vi "Main_Stop_Global.vi"() -> ()   [LabVIEW 2016]
panel:
  in  "Main_Stop":bool
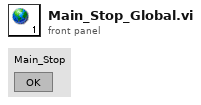
[diagram p1: front panel]
diagram:
